vi "eip tag type to tag bus type.vi"(11 "eip tag types":T2) -> (3 "data type":T1)   [LabVIEW 2013, in "EIP Tags Configuration.lvclass"]
uses:
  EIP Tags Configuration.lvclass
  eip tag types.ctl
  <vilib>/NI/Tag Bus/tag/Data Type.ctl
  <vilib>/NI/Tag Bus/tag/tag descriptor.lvclass
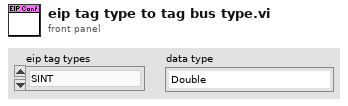
[diagram p1: front panel]
types:
  T1 = typedef "tag bus.lvlib/tag descriptor.lvclass/Data Type.ctl" = enum16{"Double", "Single", "I64", "I32", "I16", "I8", "U64", "U32", "U16", "U8", "Boolean", "String", "Array of Double", "Array of Single", "Array of I64", "Array of I32", "Array of I16", "Array of I8", "Array of U64", "Array of U32", "Array of U16", "Array of U8", "Array of Boolean", "Array of String"}
  T2 = typedef "EIP Tags Configuration.lvclass/eip tag types.ctl" = enum16{"SINT", "INT", "DINT", "REAL", "BOOL", "STRING"}
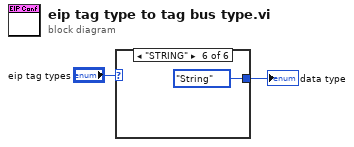
[diagram p0: block diagram]
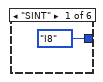
[diagram p2: hidden frame]
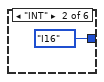
[diagram p3: hidden frame]
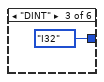
[diagram p4: hidden frame]
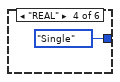
[diagram p5: hidden frame]
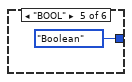
[diagram p6: hidden frame]
diagram:
  n1 = case shown="\"STRING\"" "eip tag types" {
    tunnel: [Data_Type."I8" ("data type") Data_Type."I16" ("data type") Data_Type."I32" ("data type") Data_Type."Single" ("data type") Data_Type."Boolean" ("data type") Data_Type."String" ("data type")] -> w1
    frame "SINT" {
    }
    frame "INT" {
    }
    frame "DINT" {
    }
    frame "REAL" {
    }
    frame "BOOL" {
    }
    frame "STRING" {
    }
  }
  "data type" <- w1
